vi "Estrutura-1.vi"() -> ()   [LabVIEW 2014]
doc: "André Romero - 2016\nandretec@ifsc.usp.br\nIFSC - USP"
panel:
  in  "Zera Motor":bool
  out "stop":bool
  out "GetPOS X":dbl=3.3289995335820897 format="%#_6f"
  out "GetPOS Y":dbl=2.244140625 format="%_6f"
  in  "Graph X":dbl[](array[numeric])=[0.0, 0.0, 3.334217583955224, 3.334217583955224, 3.334217583955224, 3.334217583955224, 3.334217583955224, 3.4341767723880596, 3.4341767723880596, 3.4341767723880596, 3.4341767723880596, 3.4341767723880596, 3.6537721548507465, 3.6537721548507465, 3.6537721548507465, 3.6537721548507465, 3.6537721548507465, 3.904267723880597, 3.904267723880597, 3.904267723880597, 3.904267723880597, 3.904267723880597, 4.148554104477612, 4.148554104477612, 4.148554104477612, 4.148554104477612, 4.148554104477612, 4.2985949160447765, 4.2985949160447765, 4.2985949160447765, 4.2985949160447765, 4.2985949160447765, 4.328970382462686, 4.328970382462686, 4.328970382462686, 4.328970382462686, 4.328970382462686, 4.328970382462686, 4.328970382462686, 4.328970382462686, 4.328882929104478, 4.328882929104478, 4.328882929104478, 4.328882929104478, 4.328882929104478, 4.393423507462686, 4.393423507462686, 4.393423507462686, 4.393423507462686, 4.393423507462686, 4.538071361940299, 4.538071361940299, 4.538071361940299, 4.538071361940299, 4.538071361940299, 4.578999533582089, 4.578999533582089, 4.578999533582089, 4.578999533582089, 4.578999533582089, 4.578999533582089, 4.578999533582089, 4.578970382462686, 4.578970382462686, 4.578970382462686, 4.578970382462686, 4.578970382462686, 4.5974230410447765, 4.5974230410447765, 4.5974230410447765, 4.5974230410447765, 4.5974230410447765, 4.728486473880597, 4.728486473880597, 4.728486473880597, 4.728486473880597, 4.728486473880597, 4.947382229477612, 4.947382229477612, 4.947382229477612, 4.947382229477612, 4.947382229477612, 5.066435401119403, 5.066435401119403, 5.066435401119403, 5.066435401119403, 5.066435401119403, 5.078999533582089, 5.078999533582089, 5.078999533582089, 5.078999533582089, 5.078999533582089, 5.078999533582089, 5.078999533582089, 5.078999533582089, 5.078941231343284, 5.078941231343284, 5.078941231343284, 5.078941231343284, 5.078941231343284, 5.1449102145522385, 5.1449102145522385, 5.1449102145522385, 5.1449102145522385, 5.1449102145522385, 5.225163246268656, 5.225163246268656, 5.225163246268656, 5.225163246268656, 5.225163246268656, 5.520464085820896, 5.520464085820896, 5.520464085820896, 5.520464085820896, 5.520464085820896, 5.578999533582089, 5.578999533582089, 5.578999533582089, 5.578999533582089, 5.578999533582089, 5.578970382462686, 5.578970382462686, 5.578970382462686, 5.578970382462686, 5.578970382462686, 5.578970382462686, 5.578970382462686, 5.578941231343284, 5.578941231343284, 5.578941231343284, 5.578941231343284, 5.578941231343284, 5.6462511660447765, 5.6462511660447765, 5.6462511660447765, 5.6462511660447765, 5.6462511660447765, 5.839144123134329, 5.839144123134329, 5.839144123134329, 5.839144123134329, 5.839144123134329, 5.945953824626866, 5.945953824626866, 5.945953824626866, 5.945953824626866, 5.945953824626866, 6.078999533582089, 6.078999533582089, 6.078999533582089, 6.078999533582089, 6.078999533582089, 6.078941231343284, 6.078941231343284, 6.078941231343284, 6.078941231343284, 6.078941231343284, 6.078941231343284, 6.078941231343284, 6.078941231343284, 6.078912080223881, 6.078912080223881, 6.078912080223881, 6.078912080223881, 6.078912080223881, 6.096052938432836, 6.096052938432836, 6.096052938432836, 6.096052938432836, 6.096052938432836, 6.224580223880597, 6.224580223880597, 6.224580223880597, 6.224580223880597, 6.224580223880597, 6.520143423507463, 6.520143423507463, 6.520143423507463, 6.520143423507463, 6.520143423507463, 6.565181902985074, 6.565181902985074, 6.565181902985074, 6.565181902985074, 6.565181902985074, 6.578970382462686, 6.578970382462686, 6.578970382462686, 6.578970382462686, 6.578970382462686, 6.578970382462686, 6.578970382462686, 6.578941231343284, 6.578941231343284, 6.578941231343284, 6.578941231343284, 6.578941231343284, 6.646280317164179, 6.646280317164179, 6.646280317164179, 6.646280317164179, 6.646280317164179, 6.839114972014926, 6.839114972014926, 6.839114972014926, 6.839114972014926, 6.839114972014926, 7.021659281716418, 7.021659281716418, 7.021659281716418, 7.021659281716418, 7.021659281716418, 7.078999533582089, 7.078999533582089, 7.078999533582089, 7.078999533582089, 7.078999533582089, 7.078970382462686, 7.078970382462686, 7.078970382462686, 7.078970382462686, 7.078970382462686, 7.078970382462686, 7.078970382462686, 7.078912080223881, 7.078912080223881, 7.078912080223881, 7.078912080223881, 7.078912080223881, 7.095848880597015, 7.095848880597015, 7.095848880597015, 7.095848880597015, 7.095848880597015, 7.224055503731344, 7.224055503731344, 7.224055503731344, 7.224055503731344, 7.224055503731344, 7.443330223880597, 7.443330223880597, 7.443330223880597, 7.443330223880597, 7.443330223880597, 7.56503614738806, 7.56503614738806, 7.56503614738806, 7.56503614738806, 7.56503614738806, 7.578970382462686, 7.578970382462686, 7.578970382462686, 7.578970382462686, 7.578970382462686, 7.578970382462686, 7.578970382462686, 7.578970382462686, 7.578912080223881, 7.578912080223881, 7.578912080223881, 7.578912080223881, 7.578912080223881, 7.646047108208955, 7.646047108208955, 7.646047108208955, 7.646047108208955, 7.646047108208955, 7.789995335820896, 7.789995335820896, 7.789995335820896, 7.789995335820896, 7.789995335820896, 7.829028684701493, 7.829028684701493, 7.829028684701493, 7.829028684701493, 7.829028684701493, 7.829028684701493, 7.829028684701493, 7.829028684701493, 7.842409048507463, 7.842409048507463, 7.842409048507463, 7.842409048507463, 7.842409048507463, 7.963444496268656, 7.963444496268656, 7.963444496268656, 7.963444496268656, 7.963444496268656, 8.070837220149254, 8.070837220149254, 8.070837220149254, 8.070837220149254, 8.070837220149254, 8.446274486940299, 8.446274486940299, 8.446274486940299, 8.446274486940299, 8.446274486940299, 8.682660914179104, 8.682660914179104, 8.682660914179104, 8.682660914179104, 8.682660914179104, 8.762826492537313, 8.762826492537313, 8.762826492537313, 8.762826492537313, 8.762826492537313, 8.829028684701493, 8.829028684701493, 8.829028684701493, 8.829028684701493, 8.829028684701493, 8.829028684701493, 8.829028684701493, 8.829028684701493, 8.829028684701493, 8.829028684701493, 8.829028684701493, 8.829028684701493, 8.829028684701493, 8.829028684701493, 8.829028684701493, 8.829028684701493, 8.829028684701493, 8.829028684701493, 8.829028684701493, 8.829028684701493, 8.829028684701493, 8.829028684701493, 8.829028684701493, 8.829028684701493, 8.829028684701493, 8.829028684701493, 8.829028684701493, 8.829028684701493, 8.829028684701493, 8.829028684701493, 8.829028684701493, 8.829028684701493, 8.829028684701493, 8.829028684701493, 8.829028684701493, 8.829028684701493, 8.829028684701493, 8.829028684701493, 8.829028684701493, 8.829028684701493, 8.829028684701493, 8.829028684701493, 8.828970382462687, 8.828970382462687, 8.828970382462687, 8.828970382462687, 8.828970382462687, 8.763671875, 8.763671875, 8.763671875, 8.763671875, 8.763671875, 8.684235074626866, 8.684235074626866, 8.684235074626866, 8.684235074626866, 8.684235074626866, 8.44805270522388, 8.44805270522388, 8.44805270522388, 8.44805270522388, 8.44805270522388, 8.072527985074627, 8.072527985074627, 8.072527985074627, 8.072527985074627, 8.072527985074627, 7.958984375, 7.958984375, 7.958984375, 7.958984375, 7.958984375, 7.824335354477612, 7.824335354477612, 7.824335354477612, 7.824335354477612, 7.824335354477612, 7.828999533582089, 7.828999533582089, 7.828999533582089, 7.828999533582089, 7.828999533582089, 7.828970382462686, 7.828970382462686, 7.828970382462686, 7.828970382462686, 7.828970382462686, 7.828970382462686, 7.828970382462686, 7.828970382462686, 7.828970382462686, 7.828970382462686, 7.828970382462686, 7.828970382462686, 7.828970382462686, 7.761398087686567, 7.761398087686567, 7.761398087686567, 7.761398087686567, 7.761398087686567, 7.607334421641791, 7.607334421641791, 7.607334421641791, 7.607334421641791, 7.607334421641791, 7.554075326492537, 7.554075326492537, 7.554075326492537, 7.554075326492537, 7.554075326492537, 7.578999533582089, 7.578999533582089, 7.578999533582089, 7.578999533582089, 7.578999533582089, 7.578999533582089, 7.578999533582089, 7.578999533582089, 7.578999533582089, 7.578999533582089, 7.578999533582089, 7.578999533582089, 7.578970382462686, 7.578970382462686, 7.578970382462686, 7.578970382462686, 7.578970382462686, 7.561887826492537, 7.561887826492537, 7.561887826492537, 7.561887826492537, 7.561887826492537, 7.433652052238806, 7.433652052238806, 7.433652052238806, 7.433652052238806, 7.433652052238806, 7.20869286380597, 7.20869286380597, 7.20869286380597, 7.20869286380597, 7.20869286380597, 7.074306203358209, 7.074306203358209, 7.074306203358209, 7.074306203358209, 7.074306203358209, 7.065181902985074, 7.065181902985074, 7.065181902985074, 7.065181902985074, 7.065181902985074, 7.078970382462686, 7.078970382462686, 7.078970382462686, 7.078970382462686, 7.078970382462686, 7.078970382462686, 7.078970382462686, 7.078970382462686, 7.078970382462686, 7.078970382462686, 7.078970382462686, 7.078970382462686, 7.062674906716418, 7.062674906716418, 7.062674906716418, 7.062674906716418, 7.062674906716418, 6.935459421641791, 6.935459421641791, 6.935459421641791, 6.935459421641791, 6.935459421641791, 6.710500233208955, 6.710500233208955, 6.710500233208955, 6.710500233208955, 6.710500233208955, 6.575005830223881, 6.575005830223881, 6.575005830223881, 6.575005830223881, 6.575005830223881, 6.564802938432836, 6.564802938432836, 6.564802938432836, 6.564802938432836, 6.564802938432836, 6.564802938432836, 6.578970382462686, 6.578970382462686, 6.578970382462686, 6.578970382462686, 6.578970382462686, 6.578970382462686, 6.578970382462686, 6.578970382462686, 6.578970382462686, 6.578970382462686, 6.578970382462686, 6.578970382462686, 6.511747901119403, 6.511747901119403, 6.511747901119403, 6.511747901119403, 6.511747901119403, 6.430795242537314, 6.430795242537314, 6.430795242537314, 6.430795242537314, 6.430795242537314, 6.2057486007462686, 6.2057486007462686, 6.2057486007462686, 6.2057486007462686, 6.2057486007462686, 6.05410447761194, 6.05410447761194, 6.05410447761194, 6.05410447761194, 6.05410447761194, 6.066143889925373, 6.066143889925373, 6.066143889925373, 6.066143889925373, 6.066143889925373, 6.078970382462686, 6.078970382462686, 6.078970382462686, 6.078970382462686, 6.078970382462686, 6.078970382462686, 6.078970382462686, 6.078970382462686, 6.078970382462686, 6.078970382462686, 6.078970382462686, 6.078970382462686, 6.078970382462686, 6.012534981343284, 6.012534981343284, 6.012534981343284, 6.012534981343284, 6.012534981343284, 5.932252798507463, 5.932252798507463, 5.932252798507463, 5.932252798507463, 5.932252798507463, 5.7072644589552235, 5.7072644589552235, 5.7072644589552235, 5.7072644589552235, 5.7072644589552235, 5.554191930970149, 5.554191930970149, 5.554191930970149, 5.554191930970149, 5.554191930970149, 5.5657357742537314, 5.5657357742537314, 5.5657357742537314, 5.5657357742537314, 5.5657357742537314, 5.578970382462686, 5.578970382462686, 5.578970382462686, 5.578970382462686, 5.578970382462686, 5.578970382462686, 5.578970382462686, 5.578970382462686, 5.578970382462686, 5.578970382462686, 5.578970382462686, 5.578970382462686, 5.513467817164179, 5.513467817164179, 5.513467817164179, 5.513467817164179, 5.513467817164179, 5.433535447761194, 5.433535447761194, 5.433535447761194, 5.433535447761194, 5.433535447761194, 5.125757929104478, 5.125757929104478, 5.125757929104478, 5.125757929104478, 5.125757929104478, 5.054279384328358, 5.054279384328358, 5.054279384328358, 5.054279384328358, 5.054279384328358, 5.065269356343284, 5.065269356343284, 5.065269356343284, 5.065269356343284, 5.065269356343284, 5.078999533582089, 5.078999533582089, 5.078999533582089, 5.078999533582089, 5.078999533582089, 5.078999533582089, 5.078999533582089, 5.078999533582089, 5.078970382462686, 5.078970382462686, 5.078970382462686, 5.078970382462686, 5.078970382462686, 5.014663013059701, 5.014663013059701, 5.014663013059701, 5.014663013059701, 5.014663013059701, 4.9351679104477615, 4.9351679104477615, 4.9351679104477615, 4.9351679104477615, 4.9351679104477615, 4.710062966417911, 4.710062966417911, 4.710062966417911, 4.710062966417911, 4.710062966417911, 4.554250233208955, 4.554250233208955, 4.554250233208955, 4.554250233208955, 4.554250233208955, 4.5648320895522385, 4.5648320895522385, 4.5648320895522385, 4.5648320895522385, 4.5648320895522385, 4.578970382462686, 4.578970382462686, 4.578970382462686, 4.578970382462686, 4.578970382462686, 4.578970382462686, 4.578970382462686, 4.578970382462686, 4.578970382462686, 4.578970382462686, 4.578970382462686, 4.578970382462686, 4.511864505597015, 4.511864505597015, 4.511864505597015, 4.511864505597015, 4.511864505597015, 4.357771688432836, 4.357771688432836, 4.357771688432836, 4.357771688432836, 4.357771688432836, 4.315269356343284, 4.315269356343284, 4.315269356343284, 4.315269356343284, 4.315269356343284, 4.328999533582089, 4.328999533582089, 4.328999533582089, 4.328999533582089, 4.328999533582089, 4.328970382462686, 4.328970382462686, 4.328970382462686, 4.328970382462686, 4.328970382462686, 4.328970382462686, 4.328970382462686, 4.314948694029851, 4.314948694029851, 4.314948694029851, 4.314948694029851, 4.314948694029851, 4.269443796641791, 4.269443796641791, 4.269443796641791, 4.269443796641791, 4.269443796641791, 4.0843633395522385, 4.0843633395522385, 4.0843633395522385, 4.0843633395522385, 4.0843633395522385, 3.833955223880597, 3.833955223880597, 3.833955223880597, 3.833955223880597, 3.833955223880597, 3.583896921641791, 3.583896921641791, 3.583896921641791, 3.583896921641791, 3.583896921641791, 3.3820837220149254, 3.3820837220149254, 3.3820837220149254, 3.3820837220149254, 3.3820837220149254, 3.3048041044776117, 3.3048041044776117, 3.3048041044776117, 3.3048041044776117, 3.3048041044776117, 3.3289995335820897, 3.3289995335820897, 3.3289995335820897, 3.3289995335820897, 3.3289995335820897, 3.3289995335820897]
  in  "Graph Y":dbl[](array[numeric])=[0.0, 0.0, 1.244140625, 1.244140625, 1.244140625, 1.244140625, 1.244140625, 1.244140625, 1.244140625, 1.244140625, 1.244140625, 1.244140625, 1.244140625, 1.244140625, 1.244140625, 1.244140625, 1.244140625, 1.244140625, 1.244140625, 1.244140625, 1.244140625, 1.244140625, 1.244140625, 1.244140625, 1.244140625, 1.244140625, 1.244140625, 1.244140625, 1.244140625, 1.244140625, 1.244140625, 1.244140625, 1.244140625, 1.244140625, 1.244140625, 1.244140625, 1.244140625, 1.244140625, 1.244140625, 1.244140625, 1.2545475746268657, 1.2545475746268657, 1.2545475746268657, 1.2545475746268657, 1.2545475746268657, 1.3686742070895523, 1.3686742070895523, 1.3686742070895523, 1.3686742070895523, 1.3686742070895523, 1.4834713152985075, 1.4834713152985075, 1.4834713152985075, 1.4834713152985075, 1.4834713152985075, 1.494169776119403, 1.494169776119403, 1.494169776119403, 1.494169776119403, 1.494169776119403, 1.494169776119403, 1.494169776119403, 1.484229244402985, 1.484229244402985, 1.484229244402985, 1.484229244402985, 1.484229244402985, 1.3714727145522387, 1.3714727145522387, 1.3714727145522387, 1.3714727145522387, 1.3714727145522387, 1.1491662779850746, 1.1491662779850746, 1.1491662779850746, 1.1491662779850746, 1.1491662779850746, 0.9993003731343284, 0.9993003731343284, 0.9993003731343284, 0.9993003731343284, 0.9993003731343284, 0.974725979477612, 0.974725979477612, 0.974725979477612, 0.974725979477612, 0.974725979477612, 0.9941697761194029, 0.9941697761194029, 0.9941697761194029, 0.9941697761194029, 0.9941697761194029, 0.9941697761194029, 0.9941697761194029, 0.9941697761194029, 1.0062383395522387, 1.0062383395522387, 1.0062383395522387, 1.0062383395522387, 1.0062383395522387, 1.1240671641791045, 1.1240671641791045, 1.1240671641791045, 1.1240671641791045, 1.1240671641791045, 1.3429920708955223, 1.3429920708955223, 1.3429920708955223, 1.3429920708955223, 1.3429920708955223, 1.4750757929104477, 1.4750757929104477, 1.4750757929104477, 1.4750757929104477, 1.4750757929104477, 1.4941989272388059, 1.4941989272388059, 1.4941989272388059, 1.4941989272388059, 1.4941989272388059, 1.494140625, 1.494140625, 1.494140625, 1.494140625, 1.494140625, 1.494140625, 1.494140625, 1.4831215018656716, 1.4831215018656716, 1.4831215018656716, 1.4831215018656716, 1.4831215018656716, 1.3673624067164178, 1.3673624067164178, 1.3673624067164178, 1.3673624067164178, 1.3673624067164178, 1.144502098880597, 1.144502098880597, 1.144502098880597, 1.144502098880597, 1.144502098880597, 0.9972889458955224, 0.9972889458955224, 0.9972889458955224, 0.9972889458955224, 0.9972889458955224, 0.9756879664179104, 0.9756879664179104, 0.9756879664179104, 0.9756879664179104, 0.9756879664179104, 0.9941697761194029, 0.9941697761194029, 0.9941697761194029, 0.9941697761194029, 0.9941697761194029, 0.9941697761194029, 0.9941697761194029, 0.9941697761194029, 1.0047224813432836, 1.0047224813432836, 1.0047224813432836, 1.0047224813432836, 1.0047224813432836, 1.1194612873134329, 1.1194612873134329, 1.1194612873134329, 1.1194612873134329, 1.1194612873134329, 1.3375991138059702, 1.3375991138059702, 1.3375991138059702, 1.3375991138059702, 1.3375991138059702, 1.4731518190298507, 1.4731518190298507, 1.4731518190298507, 1.4731518190298507, 1.4731518190298507, 1.4941989272388059, 1.4941989272388059, 1.4941989272388059, 1.4941989272388059, 1.4941989272388059, 1.494140625, 1.494140625, 1.494140625, 1.494140625, 1.494140625, 1.494140625, 1.494140625, 1.482771688432836, 1.482771688432836, 1.482771688432836, 1.482771688432836, 1.482771688432836, 1.3662838152985075, 1.3662838152985075, 1.3662838152985075, 1.3662838152985075, 1.3662838152985075, 1.1431319962686568, 1.1431319962686568, 1.1431319962686568, 1.1431319962686568, 1.1431319962686568, 0.9968808302238806, 0.9968808302238806, 0.9968808302238806, 0.9968808302238806, 0.9968808302238806, 0.9758920242537313, 0.9758920242537313, 0.9758920242537313, 0.9758920242537313, 0.9758920242537313, 0.9941697761194029, 0.9941697761194029, 0.9941697761194029, 0.9941697761194029, 0.9941697761194029, 0.9941697761194029, 0.9941697761194029, 1.0045475746268657, 1.0045475746268657, 1.0045475746268657, 1.0045475746268657, 1.0045475746268657, 1.1187616604477613, 1.1187616604477613, 1.1187616604477613, 1.1187616604477613, 1.1187616604477613, 1.3368703358208955, 1.3368703358208955, 1.3368703358208955, 1.3368703358208955, 1.3368703358208955, 1.4729477611940298, 1.4729477611940298, 1.4729477611940298, 1.4729477611940298, 1.4729477611940298, 1.4941989272388059, 1.4941989272388059, 1.4941989272388059, 1.4941989272388059, 1.4941989272388059, 1.494140625, 1.494140625, 1.494140625, 1.494140625, 1.494140625, 1.494140625, 1.494140625, 1.494140625, 1.4824801772388059, 1.4824801772388059, 1.4824801772388059, 1.4824801772388059, 1.4824801772388059, 1.365467583955224, 1.365467583955224, 1.365467583955224, 1.365467583955224, 1.365467583955224, 1.236677938432836, 1.236677938432836, 1.236677938432836, 1.236677938432836, 1.236677938432836, 1.2328591417910448, 1.2328591417910448, 1.2328591417910448, 1.2328591417910448, 1.2328591417910448, 1.2328591417910448, 1.2328591417910448, 1.2328591417910448, 1.2328591417910448, 1.2328591417910448, 1.2328591417910448, 1.2328591417910448, 1.2328591417910448, 1.2328591417910448, 1.2328591417910448, 1.2328591417910448, 1.2328591417910448, 1.2328591417910448, 1.2328591417910448, 1.2328591417910448, 1.2328591417910448, 1.2328591417910448, 1.2328591417910448, 1.2328591417910448, 1.2328591417910448, 1.2328591417910448, 1.2328591417910448, 1.2328591417910448, 1.2328591417910448, 1.2328591417910448, 1.2328591417910448, 1.2328591417910448, 1.2328591417910448, 1.2328591417910448, 1.2328591417910448, 1.2328591417910448, 1.2328591417910448, 1.2328591417910448, 1.2328591417910448, 1.2328591417910448, 1.2328591417910448, 1.2328591417910448, 1.2328591417910448, 1.2328591417910448, 1.2328591417910448, 1.254256063432836, 1.254256063432836, 1.254256063432836, 1.254256063432836, 1.254256063432836, 1.3677122201492538, 1.3677122201492538, 1.3677122201492538, 1.3677122201492538, 1.3677122201492538, 1.5961986940298507, 1.5961986940298507, 1.5961986940298507, 1.5961986940298507, 1.5961986940298507, 1.8465776585820894, 1.8465776585820894, 1.8465776585820894, 1.8465776585820894, 1.8465776585820894, 2.0861998600746268, 2.0861998600746268, 2.0861998600746268, 2.0861998600746268, 2.0861998600746268, 2.222743703358209, 2.222743703358209, 2.222743703358209, 2.222743703358209, 2.222743703358209, 2.244228078358209, 2.244228078358209, 2.244228078358209, 2.244228078358209, 2.244228078358209, 2.244140625, 2.244140625, 2.244140625, 2.244140625, 2.244140625, 2.244140625, 2.244140625, 2.244140625, 2.244140625, 2.244140625, 2.244140625, 2.244140625, 2.244140625, 2.244140625, 2.244140625, 2.244140625, 2.244140625, 2.244140625, 2.244140625, 2.244140625, 2.244140625, 2.244140625, 2.244140625, 2.244140625, 2.244140625, 2.244140625, 2.244140625, 2.244140625, 2.244140625, 2.244140625, 2.244140625, 2.244140625, 2.244140625, 2.244140625, 2.244140625, 2.244140625, 2.244140625, 2.244140625, 2.244140625, 2.244140625, 2.244140625, 2.244140625, 2.244140625, 2.244140625, 2.244140625, 2.244140625, 2.244140625, 2.244140625, 2.255451259328358, 2.255451259328358, 2.255451259328358, 2.255451259328358, 2.255451259328358, 2.371414412313433, 2.371414412313433, 2.371414412313433, 2.371414412313433, 2.371414412313433, 2.484287546641791, 2.484287546641791, 2.484287546641791, 2.484287546641791, 2.484287546641791, 2.494169776119403, 2.494169776119403, 2.494169776119403, 2.494169776119403, 2.494169776119403, 2.494140625, 2.494140625, 2.494140625, 2.494140625, 2.494140625, 2.494140625, 2.494140625, 2.494140625, 2.494140625, 2.494140625, 2.494140625, 2.494140625, 2.4838794309701493, 2.4838794309701493, 2.4838794309701493, 2.4838794309701493, 2.4838794309701493, 2.3702192164179103, 2.3702192164179103, 2.3702192164179103, 2.3702192164179103, 2.3702192164179103, 2.1474172108208953, 2.1474172108208953, 2.1474172108208953, 2.1474172108208953, 2.1474172108208953, 1.9986007462686568, 1.9986007462686568, 1.9986007462686568, 1.9986007462686568, 1.9986007462686568, 1.9750757929104477, 1.9750757929104477, 1.9750757929104477, 1.9750757929104477, 1.9750757929104477, 1.994169776119403, 1.994169776119403, 1.994169776119403, 1.994169776119403, 1.994169776119403, 1.994140625, 1.994140625, 1.994140625, 1.994140625, 1.994140625, 1.994140625, 1.994140625, 2.005859375, 2.005859375, 2.005859375, 2.005859375, 2.005859375, 2.122988572761194, 2.122988572761194, 2.122988572761194, 2.122988572761194, 2.122988572761194, 2.341592817164179, 2.341592817164179, 2.341592817164179, 2.341592817164179, 2.341592817164179, 2.474521921641791, 2.474521921641791, 2.474521921641791, 2.474521921641791, 2.474521921641791, 2.494198927238806, 2.494198927238806, 2.494198927238806, 2.494198927238806, 2.494198927238806, 2.494140625, 2.494140625, 2.494140625, 2.494140625, 2.494140625, 2.494140625, 2.494140625, 2.494140625, 2.494140625, 2.494140625, 2.494140625, 2.494140625, 2.494140625, 2.4834130130597014, 2.4834130130597014, 2.4834130130597014, 2.4834130130597014, 2.4834130130597014, 2.3685576026119404, 2.3685576026119404, 2.3685576026119404, 2.3685576026119404, 2.3685576026119404, 2.1456972947761193, 2.1456972947761193, 2.1456972947761193, 2.1456972947761193, 2.1456972947761193, 1.9977845149253732, 1.9977845149253732, 1.9977845149253732, 1.9977845149253732, 1.9977845149253732, 1.9754839085820894, 1.9754839085820894, 1.9754839085820894, 1.9754839085820894, 1.9754839085820894, 1.994169776119403, 1.994169776119403, 1.994169776119403, 1.994169776119403, 1.994169776119403, 1.994140625, 1.994140625, 1.994140625, 1.994140625, 1.994140625, 1.994140625, 1.994140625, 1.994140625, 2.0054221082089554, 2.0054221082089554, 2.0054221082089554, 2.0054221082089554, 2.0054221082089554, 2.121501865671642, 2.121501865671642, 2.121501865671642, 2.121501865671642, 2.121501865671642, 2.339931203358209, 2.339931203358209, 2.339931203358209, 2.339931203358209, 2.339931203358209, 2.4738805970149254, 2.4738805970149254, 2.4738805970149254, 2.4738805970149254, 2.4738805970149254, 2.494198927238806, 2.494198927238806, 2.494198927238806, 2.494198927238806, 2.494198927238806, 2.494140625, 2.494140625, 2.494140625, 2.494140625, 2.494140625, 2.494140625, 2.494140625, 2.494140625, 2.494140625, 2.494140625, 2.494140625, 2.494140625, 2.4830048973880596, 2.4830048973880596, 2.4830048973880596, 2.4830048973880596, 2.4830048973880596, 2.367100046641791, 2.367100046641791, 2.367100046641791, 2.367100046641791, 2.367100046641791, 2.144064832089552, 2.144064832089552, 2.144064832089552, 2.144064832089552, 2.144064832089552, 1.9971723414179106, 1.9971723414179106, 1.9971723414179106, 1.9971723414179106, 1.9971723414179106, 1.9757754197761195, 1.9757754197761195, 1.9757754197761195, 1.9757754197761195, 1.9757754197761195, 1.994169776119403, 1.994169776119403, 1.994169776119403, 1.994169776119403, 1.994169776119403, 1.994140625, 1.994140625, 1.994140625, 1.994140625, 1.994140625, 1.994140625, 1.994140625, 1.994140625, 2.0050431436567164, 2.0050431436567164, 2.0050431436567164, 2.0050431436567164, 2.0050431436567164, 2.120539878731343, 2.120539878731343, 2.120539878731343, 2.120539878731343, 2.120539878731343, 2.3390275186567164, 2.3390275186567164, 2.3390275186567164, 2.3390275186567164, 2.3390275186567164, 2.4735599347014925, 2.4735599347014925, 2.4735599347014925, 2.4735599347014925, 2.4735599347014925, 2.494198927238806, 2.494198927238806, 2.494198927238806, 2.494198927238806, 2.494198927238806, 2.494140625, 2.494140625, 2.494140625, 2.494140625, 2.494140625, 2.494140625, 2.494140625, 2.494140625, 2.494140625, 2.494140625, 2.494140625, 2.494140625, 2.483966884328358, 2.483966884328358, 2.483966884328358, 2.483966884328358, 2.483966884328358, 2.3703649720149254, 2.3703649720149254, 2.3703649720149254, 2.3703649720149254, 2.3703649720149254, 2.238485307835821, 2.238485307835821, 2.238485307835821, 2.238485307835821, 2.238485307835821, 2.2312849813432836, 2.2312849813432836, 2.2312849813432836, 2.2312849813432836, 2.2312849813432836, 2.244169776119403, 2.244169776119403, 2.244169776119403, 2.244169776119403, 2.244169776119403, 2.244140625, 2.244140625, 2.244140625, 2.244140625, 2.244140625, 2.244140625, 2.244140625, 2.244140625, 2.244140625, 2.244140625, 2.244140625, 2.244140625, 2.244140625, 2.244140625, 2.244140625, 2.244140625, 2.244140625, 2.244140625, 2.244140625, 2.244140625, 2.244140625, 2.244140625, 2.244140625, 2.244140625, 2.244140625, 2.244140625, 2.244140625, 2.244140625, 2.244140625, 2.244140625, 2.244140625, 2.244140625, 2.244140625, 2.244140625, 2.244140625, 2.244140625, 2.244140625, 2.244140625, 2.244140625, 2.244140625, 2.244140625, 2.244140625, 2.244140625, 2.244140625, 2.244140625, 2.244140625, 2.244140625, 2.244140625]
  out "XY Graph":cluster{"Graph X":dbl[], "Graph Y":dbl[]}(graph)
  in  "Aceleração":dbl=1.0
  in  "Iniciar":bool
  in  "Velocidade":sgl=0.05
  out "Motor Y\nLigado":bool=TRUE
  out "Motor X \nLigado":bool=TRUE
  # "(mm/s)"
  # "(mm/s.s)"
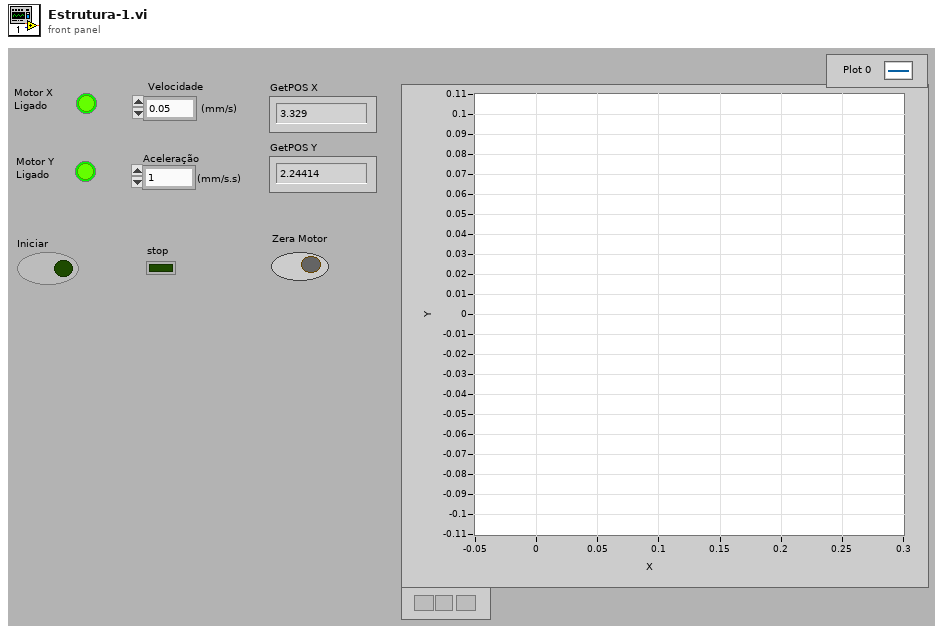
[diagram p1: front panel]
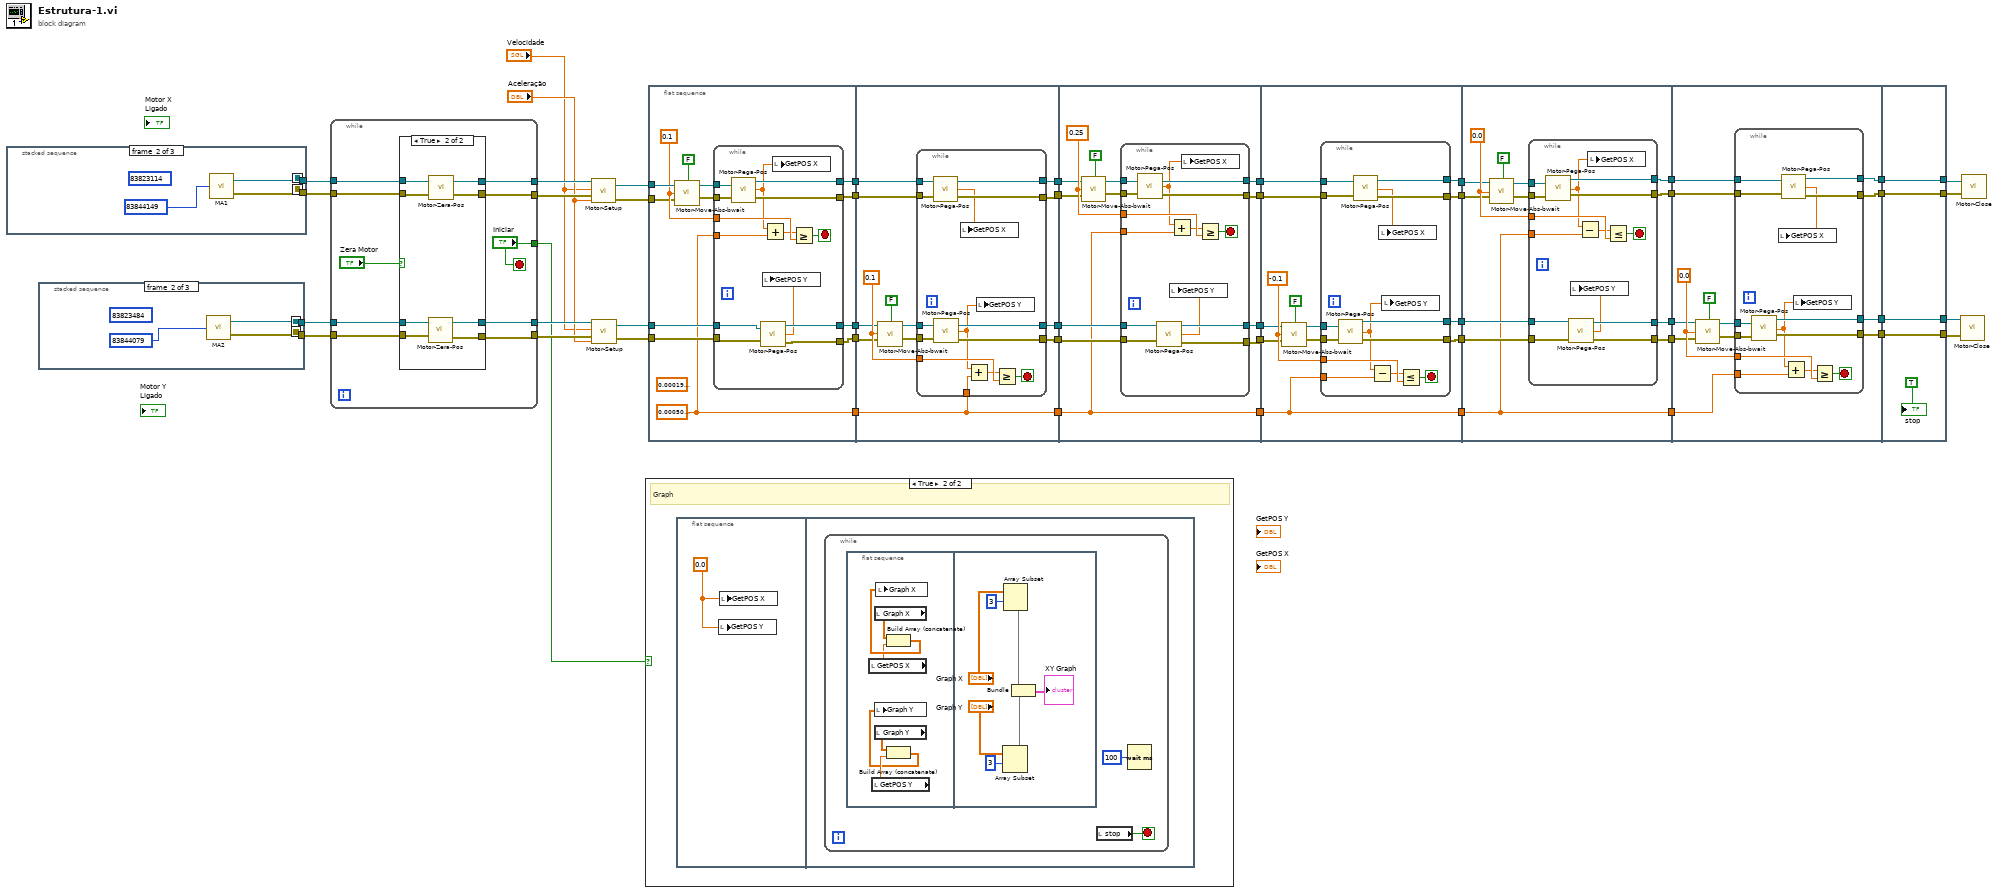
[diagram p0: block diagram]
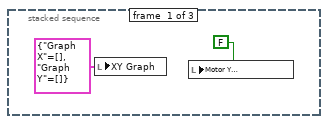
[diagram p4: hidden frame]
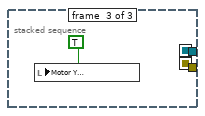
[diagram p5: hidden frame]
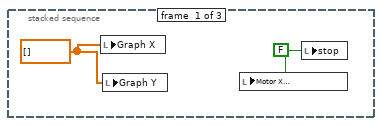
[diagram p6: hidden frame]
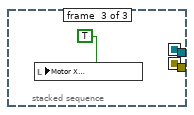
[diagram p7: hidden frame]
diagram:
  n1 = stacked-sequence {
    seq-local: [_ w53 _] -> [_ _ w56]
    seq-local: [_ w52 _] -> [_ _ w55]
    tunnel: [_ _ w56] -> w9
    tunnel: [_ _ w55] -> w8
    frame #0 {
      w49 = dbl[] []
      w50 = FALSE ("x = y?")
      n2 = local write "Graph X"(w49) -> ()
      n3 = local write "Graph Y"(w49) -> ()
      n4 = local write "Motor X \nLigado"(w50) -> ()
      n5 = local write "stop"(w50) -> ()
    }
    frame #1 {
      (unwired) 83823114 ("HWSerialNum")
      n6 = call "MA1.vi"("HWSerialNum"=83844149) -> ("MG17Motor 2"=w53:refnum<k7>, "error out"=w52:errorcluster)
    }
    frame #2 {
      n7 = local write "Motor X \nLigado"(TRUE ("x = y?")) -> ()
    }
  }
  n8 = stacked-sequence {
    seq-local: [_ w61 _] -> [_ _ w64]
    seq-local: [_ w60 _] -> [_ _ w63]
    tunnel: [_ _ w64] -> w7
    tunnel: [_ _ w63] -> w6
    frame #0 {
      n9 = local write "XY Graph"(cluster{"Graph X":dbl[], "Graph Y":dbl[]} {"Graph X"=[], "Graph Y"=[]} ("XY Graph")) -> ()
      n10 = local write "Motor Y\nLigado"(FALSE ("Motor3\nLigado")) -> ()
    }
    frame #1 {
      (unwired) 83823484 ("HWSerialNum")
      n11 = call "MA2.vi"("HWSerialNum"=83844079) -> ("MG17Motor 2"=w61:refnum<k7>, "error out"=w60:errorcluster)
    }
    frame #2 {
      n12 = local write "Motor Y\nLigado"(TRUE ("Motor3\nLigado")) -> ()
    }
  }
  n13 = while {
    tunnel: w8 -> [w71]
    tunnel: w6 -> [w69]
    tunnel: [w66] -> w48
    tunnel: [w65] -> w47
    tunnel: [w68] -> w46
    tunnel: [w67] -> w45
    tunnel: w9 -> [w72]
    tunnel: w7 -> [w70]
    tunnel: ["Iniciar"] -> w10
    stop <- "Iniciar" stop-if-true
    n14 = case shown="True" "Zera Motor" {
      tunnel: w72 -> [w78 w86]
      tunnel: w71 -> [w77 w85]
      tunnel: [w78 w84] -> w66
      tunnel: [w77 w83] -> w65
      tunnel: w70 -> [w76 w82]
      tunnel: w69 -> [w75 w81]
      tunnel: [w76 w80] -> w68
      tunnel: [w75 w79] -> w67
      frame False {
      }
      frame True {
        n15 = call "Motor-Zera-Pos.vi"("error"=w81, "MG17Motor A"=w82) -> ("error out"=w79:errorcluster, "MG17Motor out"=w80:refnum<k7>)
        n16 = call "Motor-Zera-Pos.vi"("error"=w85, "MG17Motor A"=w86) -> ("error out"=w83:errorcluster, "MG17Motor out"=w84:refnum<k7>)
      }
    }
  }
  n17 = call "Motor-Setup.vi"("Acc"="Aceleração", "Velocidade"="Velocidade", "error"=w47, "MG17Motor A"=w48) -> ("error out"=w41:errorcluster, "MG17Motor out"=w42:refnum<k7>)
  n18 = call "Motor-Setup.vi"("Acc"="Aceleração", "Velocidade"="Velocidade", "error"=w45, "MG17Motor A"=w46) -> ("error out"=w37:errorcluster, "MG17Motor out"=w39:refnum<k7>)
  n19 = case shown="True" w10 {
    frame False {
    }
    frame True {
      # "Graph"
      n20 = flat-sequence {
        frame #0 {
          w87 = 0.0
          n21 = local write "GetPOS Y"(w87) -> ()
          n22 = local write "GetPOS X"(w87) -> ()
        }
        frame #1 {
          n23 = while {
            stop <- w88 stop-if-true
            n24 = flat-sequence {
              frame #0 {
                n25 = local read "GetPOS X"() -> (w93:dbl)
                n26 = local read "GetPOS Y"() -> (w92:dbl)
                n27 = local read "Graph X"() -> (w95:dbl[])
                n28 = local read "Graph Y"() -> (w90:dbl[])
                n29 = Build Array (concatenate)(w95, w93) -> (w94:dbl[])
                n30 = local write "Graph X"(w94) -> ()
                n31 = Build Array (concatenate)(w90, w92) -> (w91:dbl[])
                n32 = local write "Graph Y"(w91) -> ()
              }
              frame #1 {
                n33 = Array Subset(array="Graph Y", index=3) -> (w96:dbl[])  [unwired: 1 in]
                n34 = Array Subset(array="Graph X", index=3) -> (w99:dbl[])  [unwired: 1 in]
                n35 = Bundle(w99, w96) -> (→"XY Graph":cluster{dbl[], dbl[]})  [unwired: 1 in]
              }
            }
            n36 = local read "stop"() -> (w88:bool)
            n37 = Wait (ms)(milliseconds to wait=u32 100) -> ()  [unwired: 1 out]
          }
        }
      }
    }
  }
  n38 = flat-sequence {
    tunnel: w42 -> [w113]
    tunnel: w41 -> [w111]
    tunnel: [w105] -> w40
    tunnel: w39 -> [w107]
    tunnel: [w104] -> w38
    tunnel: w37 -> [w106]
    tunnel: [w109] -> w35
    tunnel: [w108] -> w34
    tunnel: [w103] -> w5
    tunnel: w40 -> [w138]
    tunnel: w38 -> [w137]
    tunnel: [w132] -> w36
    tunnel: w35 -> [w134]
    tunnel: w34 -> [w133]
    tunnel: [w131] -> w33
    tunnel: [w136] -> w32
    tunnel: [w135] -> w30
    tunnel: w5 -> [w130]
    tunnel: [w130] -> w4
    tunnel: w36 -> [w165]
    tunnel: w33 -> [w164]
    tunnel: w32 -> [w160]
    tunnel: [w158] -> w31
    tunnel: w30 -> [w161]
    tunnel: [w159] -> w29
    tunnel: [w163] -> w28
    tunnel: [w162] -> w26
    tunnel: w4 -> [w157]
    tunnel: [w157] -> w3
    tunnel: w31 -> [w191]
    tunnel: w29 -> [w192]
    tunnel: w28 -> [w188]
    tunnel: [w186] -> w27
    tunnel: w26 -> [w187]
    tunnel: [w185] -> w25
    tunnel: [w190] -> w24
    tunnel: [w189] -> w23
    tunnel: w3 -> [w184]
    tunnel: [w184] -> w2
    tunnel: w27 -> [w218]
    tunnel: w25 -> [w219]
    tunnel: w24 -> [w215]
    tunnel: w23 -> [w214]
    tunnel: [w217] -> w22
    tunnel: [w216] -> w21
    tunnel: [w213] -> w20
    tunnel: [w212] -> w19
    tunnel: w2 -> [w211]
    tunnel: [w211] -> w1
    tunnel: w22 -> [w242]
    tunnel: w21 -> [w241]
    tunnel: w20 -> [w246]
    tunnel: w19 -> [w245]
    tunnel: [w240] -> w14
    tunnel: [w239] -> w13
    tunnel: [w244] -> w12
    tunnel: [w243] -> w11
    tunnel: w1 -> [w238]
    tunnel: [w266] -> w15
    tunnel: [w267] -> w16
    tunnel: [w268] -> w17
    tunnel: [w269] -> w18
    tunnel: w14 -> [w269]
    tunnel: w13 -> [w268]
    tunnel: w12 -> [w267]
    tunnel: w11 -> [w266]
    frame #0 {
      (unwired) sgl 0.0002 ("y")
      w103 = sgl 0.0005 ("y")
      w112 = 0.1
      n39 = call "Motor-Move-Abs-bwait.vi"("bWait"=FALSE, "error"=w111, "Posição"=w112, "MG17Motor A"=w113) -> ("error out"=w114:errorcluster, "MG17Motor out"=w115:refnum<k7>)
      n40 = while {
        tunnel: w115 -> [w129]
        tunnel: w114 -> [w128]
        tunnel: w112 -> [w126]
        tunnel: [w124] -> w109
        tunnel: [w123] -> w108
        tunnel: w107 -> [w121]
        tunnel: w106 -> [w120]
        tunnel: [w119] -> w105
        tunnel: [w118] -> w104
        tunnel: w103 -> [w116]
        stop <- w127 stop-if-true
        n41 = call "Motor-Pega-Pos.vi"("MG17Motor 2"=w129, "error out"=w128) -> ("MG17Motor 3"=w124:refnum<k7>, "pfPosition"=w122:sgl, "error out 2"=w123:errorcluster)
        n42 = call "Motor-Pega-Pos.vi"("MG17Motor 2"=w121, "error out"=w120) -> ("MG17Motor 3"=w119:refnum<k7>, "pfPosition"=w117:sgl, "error out 2"=w118:errorcluster)
        n43 = local write "GetPOS Y"(w117) -> ()
        n44 = Add(x=w122, y=w116) -> (x+y=w125:sgl)
        n45 = local write "GetPOS X"(w122) -> ()
        n46 = Greater Or Equal?(x=w125, y=w126) -> (x >= y?=w127:bool)
      }
    }
    frame #1 {
      w140 = 0.1
      n47 = call "Motor-Move-Abs-bwait.vi"("bWait"=FALSE, "error"=w137, "Posição"=w140, "MG17Motor A"=w138) -> ("error out"=w141:errorcluster, "MG17Motor out"=w142:refnum<k7>)
      n48 = while {
        tunnel: w142 -> [w156]
        tunnel: w141 -> [w155]
        tunnel: w140 -> [w153]
        tunnel: [w151] -> w136
        tunnel: [w150] -> w135
        tunnel: w134 -> [w148]
        tunnel: w133 -> [w147]
        tunnel: [w146] -> w132
        tunnel: [w145] -> w131
        tunnel: w130 -> [w143]
        stop <- w154 stop-if-true
        n49 = call "Motor-Pega-Pos.vi"("MG17Motor 2"=w148, "error out"=w147) -> ("MG17Motor 3"=w146:refnum<k7>, "pfPosition"=w144:sgl, "error out 2"=w145:errorcluster)
        n50 = call "Motor-Pega-Pos.vi"("MG17Motor 2"=w156, "error out"=w155) -> ("MG17Motor 3"=w150:refnum<k7>, "pfPosition"=w149:sgl, "error out 2"=w151:errorcluster)
        n51 = local write "GetPOS X"(w144) -> ()
        n52 = Add(x=w149, y=w143) -> (x+y=w152:sgl)
        n53 = local write "GetPOS Y"(w149) -> ()
        n54 = Greater Or Equal?(x=w152, y=w153) -> (x >= y?=w154:bool)
      }
    }
    frame #2 {
      w167 = 0.25
      n55 = call "Motor-Move-Abs-bwait.vi"("bWait"=FALSE, "error"=w164, "Posição"=w167, "MG17Motor A"=w165) -> ("error out"=w168:errorcluster, "MG17Motor out"=w169:refnum<k7>)
      n56 = while {
        tunnel: w169 -> [w183]
        tunnel: w168 -> [w182]
        tunnel: w167 -> [w180]
        tunnel: [w178] -> w163
        tunnel: [w177] -> w162
        tunnel: w161 -> [w175]
        tunnel: w160 -> [w174]
        tunnel: [w173] -> w159
        tunnel: [w172] -> w158
        tunnel: w157 -> [w170]
        stop <- w181 stop-if-true
        n57 = call "Motor-Pega-Pos.vi"("MG17Motor 2"=w183, "error out"=w182) -> ("MG17Motor 3"=w178:refnum<k7>, "pfPosition"=w176:sgl, "error out 2"=w177:errorcluster)
        n58 = call "Motor-Pega-Pos.vi"("MG17Motor 2"=w175, "error out"=w174) -> ("MG17Motor 3"=w173:refnum<k7>, "pfPosition"=w171:sgl, "error out 2"=w172:errorcluster)
        n59 = Add(x=w176, y=w170) -> (x+y=w179:sgl)
        n60 = local write "GetPOS Y"(w171) -> ()
        n61 = local write "GetPOS X"(w176) -> ()
        n62 = Greater Or Equal?(x=w179, y=w180) -> (x >= y?=w181:bool)
      }
    }
    frame #3 {
      w194 = -0.1
      n63 = call "Motor-Move-Abs-bwait.vi"("bWait"=FALSE, "error"=w191, "Posição"=w194, "MG17Motor A"=w192) -> ("error out"=w195:errorcluster, "MG17Motor out"=w196:refnum<k7>)
      n64 = while {
        tunnel: w196 -> [w210]
        tunnel: w195 -> [w209]
        tunnel: w194 -> [w207]
        tunnel: [w205] -> w190
        tunnel: [w204] -> w189
        tunnel: w188 -> [w202]
        tunnel: w187 -> [w201]
        tunnel: [w200] -> w186
        tunnel: [w199] -> w185
        tunnel: w184 -> [w197]
        stop <- w208 stop-if-true
        n65 = call "Motor-Pega-Pos.vi"("MG17Motor 2"=w210, "error out"=w209) -> ("MG17Motor 3"=w205:refnum<k7>, "pfPosition"=w203:sgl, "error out 2"=w204:errorcluster)
        n66 = call "Motor-Pega-Pos.vi"("MG17Motor 2"=w202, "error out"=w201) -> ("MG17Motor 3"=w200:refnum<k7>, "pfPosition"=w198:sgl, "error out 2"=w199:errorcluster)
        n67 = Subtract(x=w203, y=w197) -> (x-y=w206:sgl)
        n68 = local write "GetPOS X"(w198) -> ()
        n69 = local write "GetPOS Y"(w203) -> ()
        n70 = Less Or Equal?(x=w206, y=w207) -> (x <= y?=w208:bool)
      }
    }
    frame #4 {
      w221 = 0.0
      n71 = call "Motor-Move-Abs-bwait.vi"("bWait"=FALSE, "error"=w219, "Posição"=w221, "MG17Motor A"=w218) -> ("error out"=w222:errorcluster, "MG17Motor out"=w223:refnum<k7>)
      n72 = while {
        tunnel: w223 -> [w237]
        tunnel: w222 -> [w236]
        tunnel: w221 -> [w234]
        tunnel: [w232] -> w217
        tunnel: [w231] -> w216
        tunnel: w215 -> [w229]
        tunnel: w214 -> [w228]
        tunnel: [w227] -> w213
        tunnel: [w226] -> w212
        tunnel: w211 -> [w224]
        stop <- w235 stop-if-true
        n73 = call "Motor-Pega-Pos.vi"("MG17Motor 2"=w237, "error out"=w236) -> ("MG17Motor 3"=w232:refnum<k7>, "pfPosition"=w230:sgl, "error out 2"=w231:errorcluster)
        n74 = call "Motor-Pega-Pos.vi"("MG17Motor 2"=w229, "error out"=w228) -> ("MG17Motor 3"=w227:refnum<k7>, "pfPosition"=w225:sgl, "error out 2"=w226:errorcluster)
        n75 = local write "GetPOS Y"(w225) -> ()
        n76 = Subtract(x=w230, y=w224) -> (x-y=w233:sgl)
        n77 = local write "GetPOS X"(w230) -> ()
        n78 = Less Or Equal?(x=w233, y=w234) -> (x <= y?=w235:bool)
      }
    }
    frame #5 {
      w249 = 0.0
      n79 = call "Motor-Move-Abs-bwait.vi"("bWait"=FALSE, "error"=w245, "Posição"=w249, "MG17Motor A"=w246) -> ("error out"=w248:errorcluster, "MG17Motor out"=w247:refnum<k7>)
      n80 = while {
        tunnel: w247 -> [w264]
        tunnel: w248 -> [w263]
        tunnel: w249 -> [w261]
        tunnel: [w259] -> w244
        tunnel: [w258] -> w243
        tunnel: w242 -> [w256]
        tunnel: w241 -> [w255]
        tunnel: [w254] -> w240
        tunnel: [w253] -> w239
        tunnel: w238 -> [w251]
        stop <- w262 stop-if-true
        n81 = call "Motor-Pega-Pos.vi"("MG17Motor 2"=w264, "error out"=w263) -> ("MG17Motor 3"=w259:refnum<k7>, "pfPosition"=w257:sgl, "error out 2"=w258:errorcluster)
        n82 = call "Motor-Pega-Pos.vi"("MG17Motor 2"=w256, "error out"=w255) -> ("MG17Motor 3"=w254:refnum<k7>, "pfPosition"=w252:sgl, "error out 2"=w253:errorcluster)
        n83 = local write "GetPOS X"(w252) -> ()
        n84 = Add(x=w257, y=w251) -> (x+y=w260:sgl)
        n85 = local write "GetPOS Y"(w257) -> ()
        n86 = Greater Or Equal?(x=w260, y=w261) -> (x >= y?=w262:bool)
      }
    }
    frame #6 {
      "stop" <- TRUE ("stop")
    }
  }
  n87 = call "Motor-Close.vi"("error out"=w15, "MG17Motor 3"=w16) -> ()  [unwired: 1 in]
  n88 = call "Motor-Close.vi"("error out"=w17, "MG17Motor 3"=w18) -> ()  [unwired: 1 in]
